vi "Get Pressure Servo Valve Value.vi"(8 "error in (no error)":errorcluster, 11 "ILC Actuator Cylinder in":refnum<class "ILC Actuator Cylinder.lvclass">) -> (0 "error out":errorcluster, 2 "Value":dbl format="%.2f", 3 "ILC Actuator Cylinder out":refnum<class "ILC Actuator Cylinder.lvclass">)   [LabVIEW 2015, in "ILC Actuator Cylinder.lvclass"]
uses:
  ILC Actuator Cylinder.lvclass
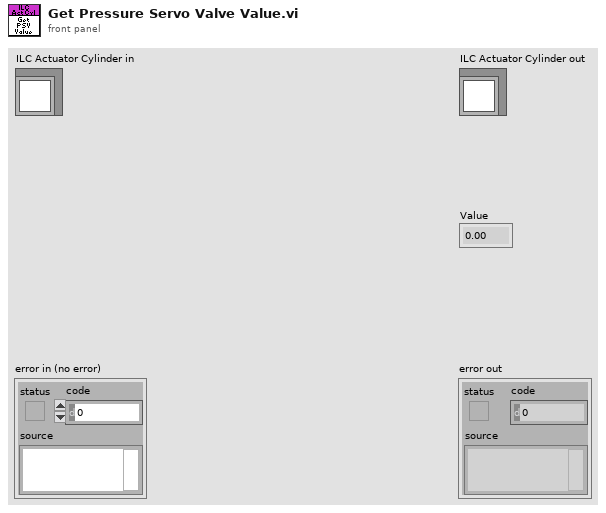
[diagram p1: front panel]
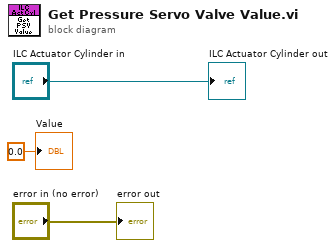
[diagram p0: block diagram]
diagram:
  "error out" <- "error in (no error)"
  "ILC Actuator Cylinder out" <- "ILC Actuator Cylinder in"
  "Value" <- 0.0 ("output")
